vi "Single_channel_mapping.vi"(11 "Channel IN":i32=16) -> (3 "Operating \nChannel(s)":bool[][](array[boolean]))   [LabVIEW 2023]
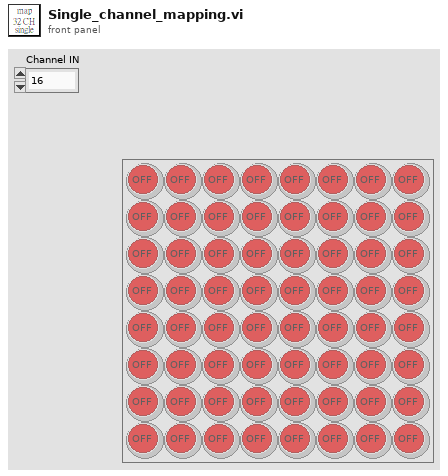
[diagram p1: front panel]
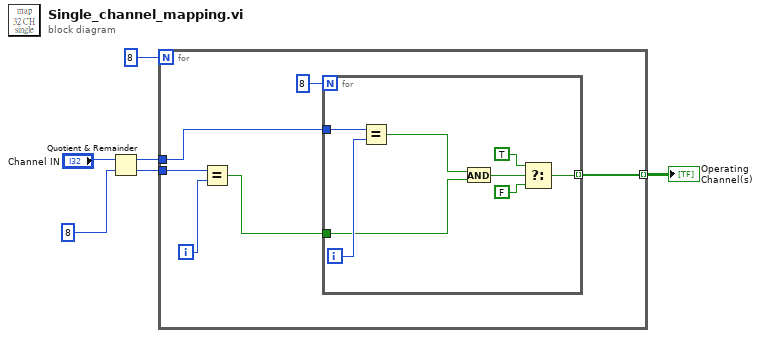
[diagram p0: block diagram]
diagram:
  n1 = Quotient & Remainder(x="Channel IN", y=8) -> (x-y*floor(x/y)=w3:i32, floor(x/y)=w2:i32)
  n2 = for {
    N: 8 -> [_]
    tunnel: [w11] -> w5 mode=indexing
    tunnel: w3 -> [w8]
    tunnel: w2 -> [w10]
    i -> [w9]
    n3 = Equal?(x=w10, y=w9) -> (x = y?=w7:bool)
    n4 = for {
      N: 8 -> [_]
      tunnel: [w15] -> w11 mode=indexing
      tunnel: w7 -> [w18]
      tunnel: w8 -> [w20]
      i -> [w19]
      n5 = Equal?(x=w20, y=w19) -> (x = y?=w13:bool)
      n6 = And(x=w13, y=w18) -> (x .and. y?=w14:bool)
      n7 = Select(t=TRUE, s=w14, f=FALSE) -> (s? t:f=w15:bool)
    }
  }
  "Operating \nChannel(s)" <- w5
